vi "Start_Client_Coms.vi"(1 "VI name to run on server":string) -> (2 "LabVIEW application reference":refnum<vi>, 3 "Checked VI name":path, 4 "Local Call":bool)   [LabVIEW 2010]
uses:
  Anemometry/Anemometry Sub Vis/Controls/App_Global.ctl
  Anemometry/Anemometry Sub Vis/Globals/Dynamic_call_global.ph.vi
panel:
  out "Application:Exported VIs In Memory":string[](array[string])
  out "IP & Port No":string
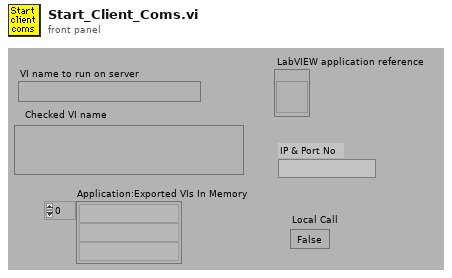
[diagram p1: front panel]
types:
  T1 = typedef "App_Global.ctl" = enum16{"Read Global", "Write to Global", "Initialise Array"}
  T2 = typedef "App_Ref_Cluster.ctl" = cluster{"Server IP & Port No":string, "Application reference":refnum<vi>}
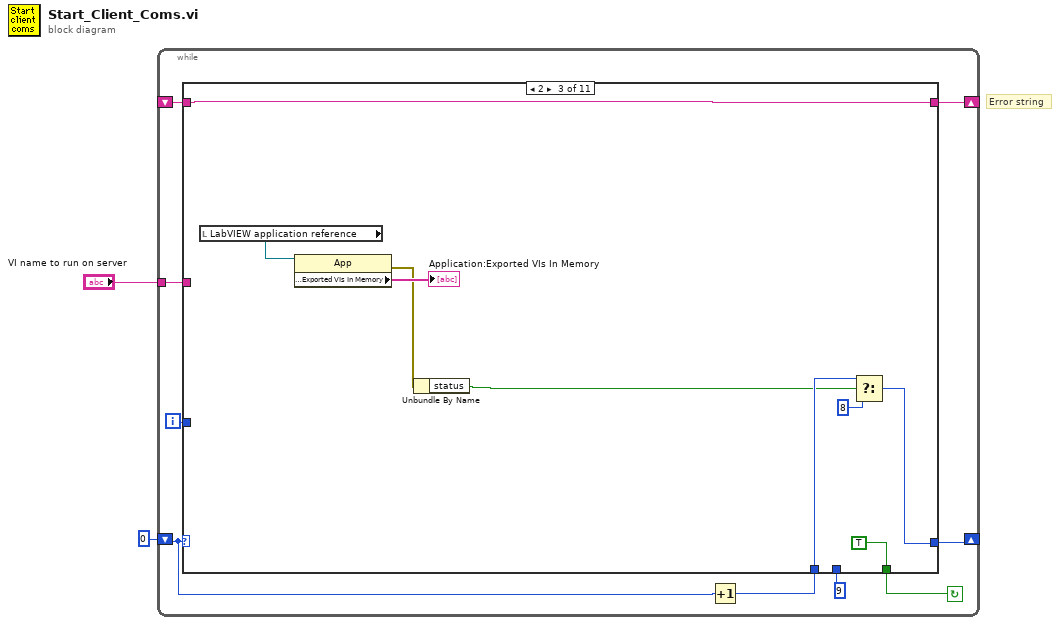
[diagram p0: block diagram]
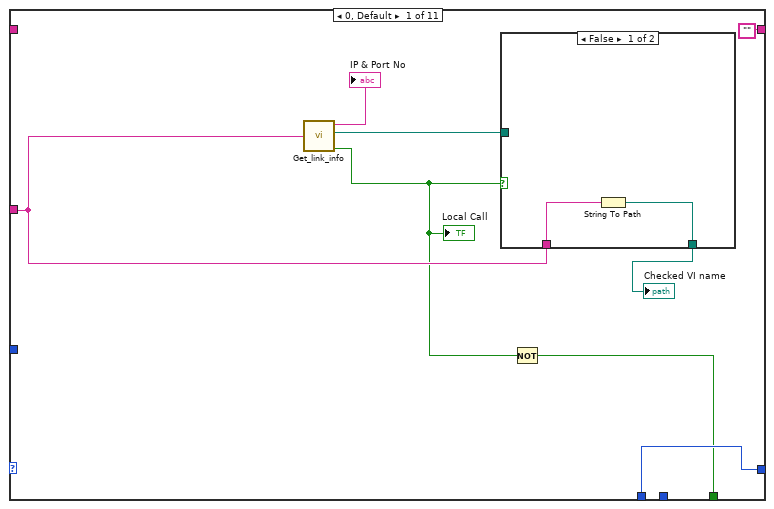
[diagram p2: hidden frame]
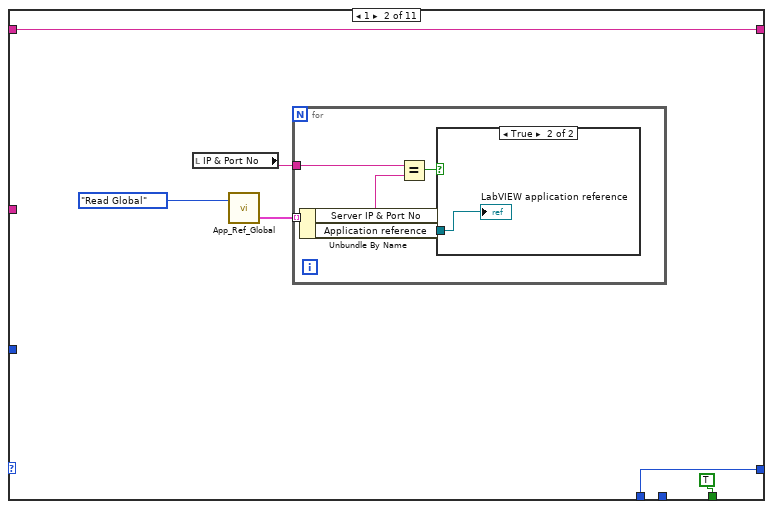
[diagram p4: hidden frame]
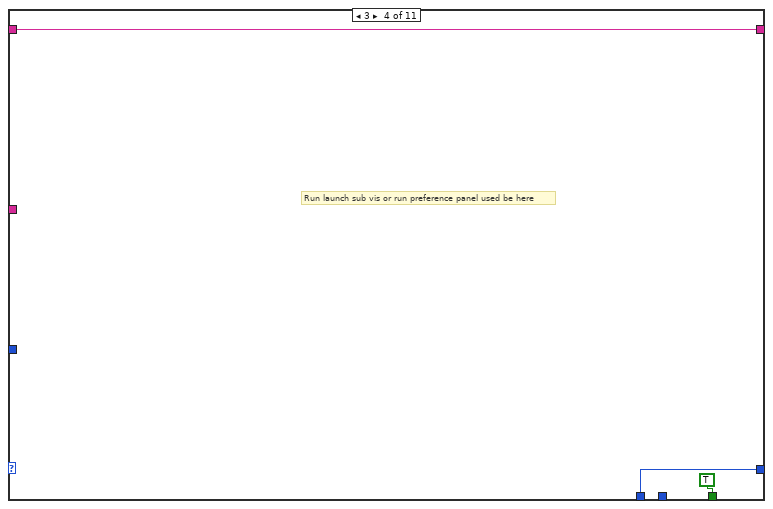
[diagram p6: hidden frame]
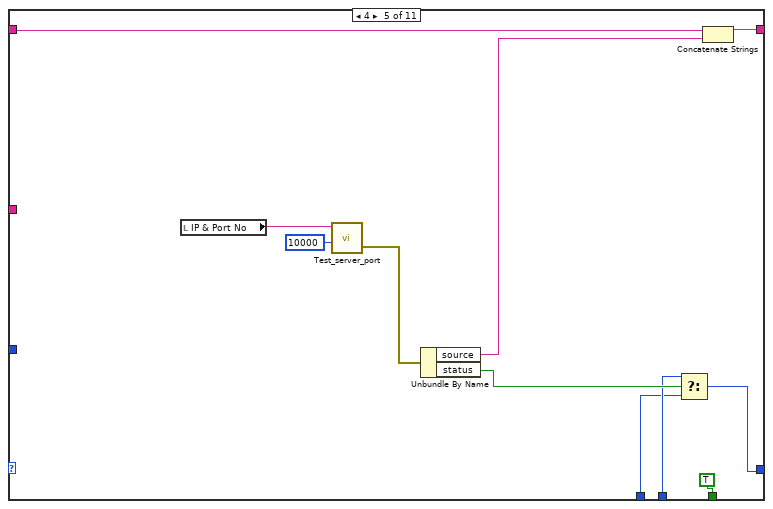
[diagram p7: hidden frame]
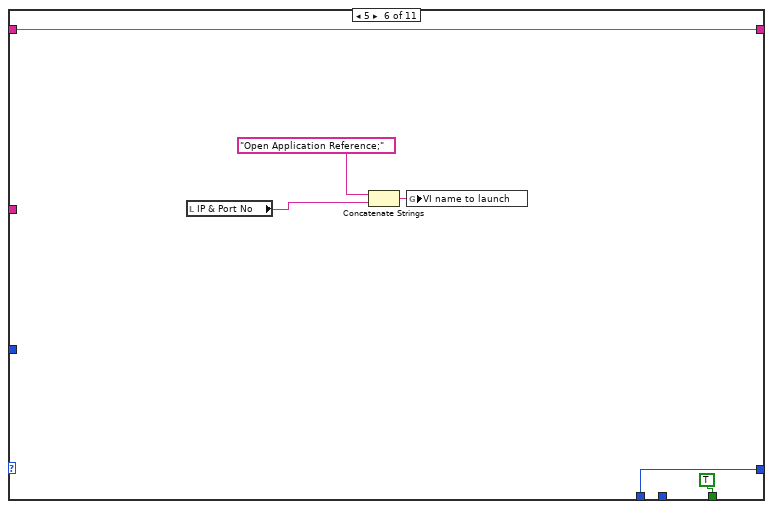
[diagram p8: hidden frame]
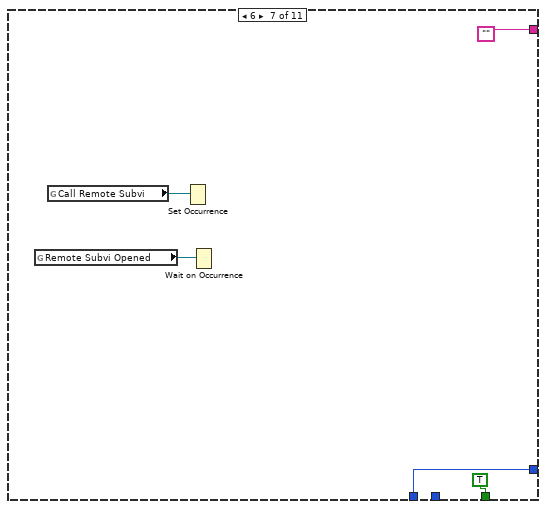
[diagram p9: hidden frame]
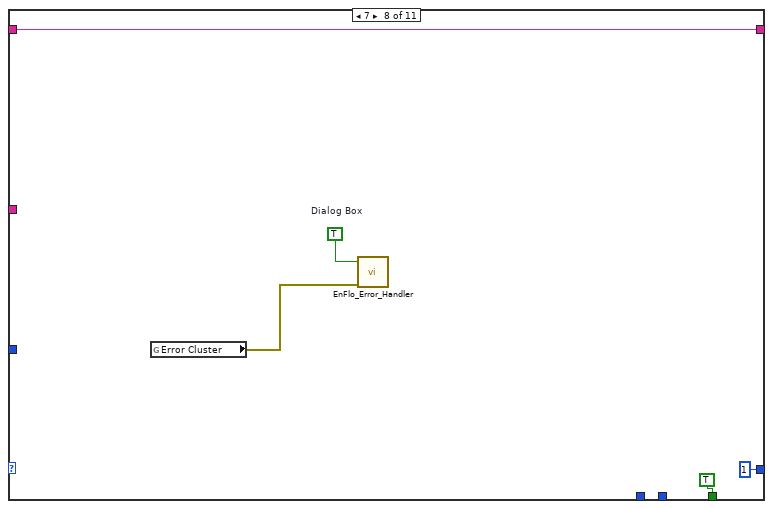
[diagram p10: hidden frame]
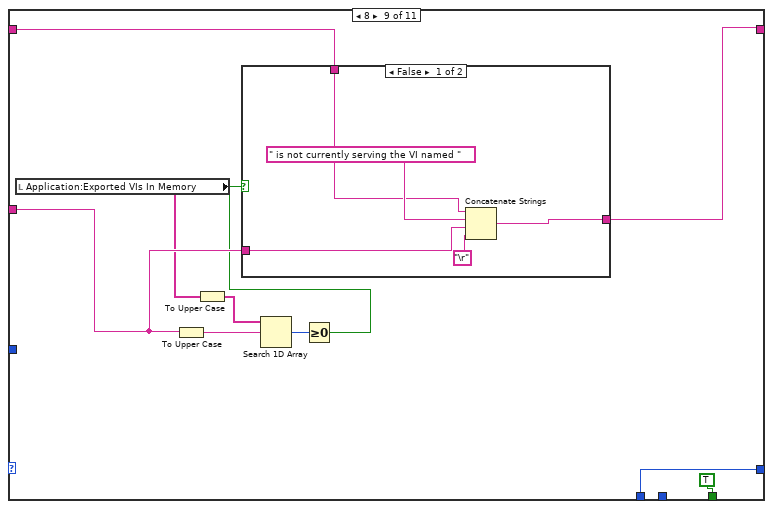
[diagram p11: hidden frame]
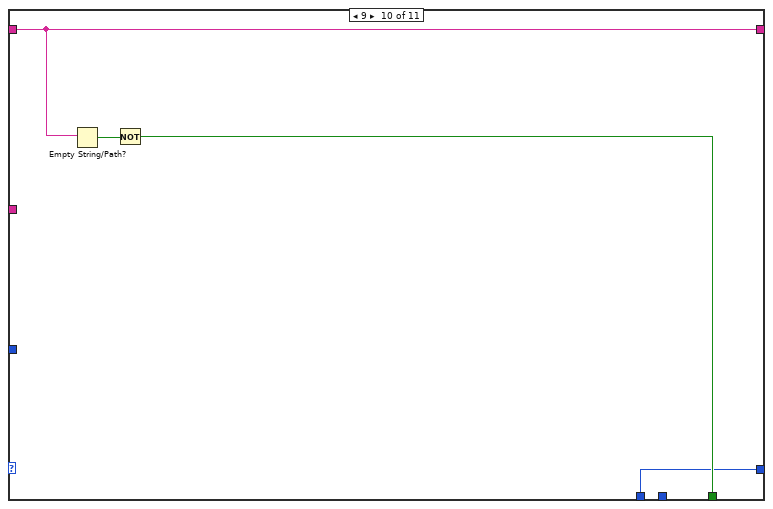
[diagram p13: hidden frame]
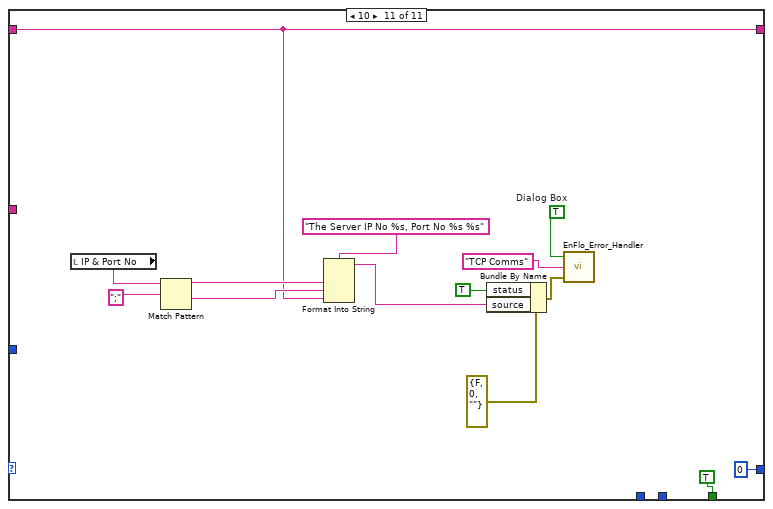
[diagram p14: hidden frame]
diagram:
  # "Error string"
  n1 = while {
    shift-left: _ -> [w4]
    shift-right: [w5] -> _
    shift-left: 0 -> [w9]
    shift-right: [w8] -> _
    tunnel: "VI name to run on server" -> [w10]
    i -> [w6]
    stop <- w11 continue-if-true
    n2 = Increment(x=w9) -> (x+1=w7:i32)
    n3 = case shown="2" w9 {
      tunnel: [w12 TRUE ("status") TRUE ("status") TRUE ("status") TRUE ("status") TRUE ("status") TRUE ("status") TRUE ("status") TRUE ("status") w92 TRUE ("status")] -> w11
      tunnel: w10 -> [w16 _ _ _ _ _ _ _ w83 _ _]
      tunnel: [w18 w26 w40 w46 w47 w62 w64 1 ("f") w76 w91 0 ("f")] -> w8
      tunnel: w7 -> [w18 w26 w41 w46 w48 w62 w64 _ w76 w91 _]
      tunnel: w6 -> [_ _ _ _ _ _ _ _ _ _ _]
      tunnel: ["" w24 w38 w44 w51 w61 "" w70 w74 w90 w98] -> w5
      tunnel: w4 -> [_ w24 w38 w44 w52 w61 _ w70 w75 w90 w98]
      tunnel: 9 ("f") -> [_ _ _ _ w49 _ _ _ _ _ _]
      frame 0, Default {
        n4 = call "Get_link_info.vi"("VI Name"=w16) -> ("Server IP & Port"=→"IP & Port No":string, "Path name"=w14:path, "Local Call?"=w13:bool)  [unwired: 1 out]
        "Local Call" <- w13
        n5 = case shown="False" w13 {
          tunnel: [w20 w22] -> w19
          tunnel: w16 -> [w21 _]
          tunnel: w14 -> [_ w22]
          frame False {
            n6 = String To Path(string=w21) -> (path=w20:path)
          }
          frame True {
          }
        }
        "Checked VI name" <- w19
        n7 = Not(x=w13) -> (.not. x?=w12:bool)
      }
      frame 1 {
        n8 = local read "IP & Port No"() -> (w27:string)
        n9 = call "App_Ref_Global.vi"("Mode"=App_Global."Read Global") -> ("Output Array"=w28:T2[])  [unwired: 1 in, 1 out]
        n10 = for {
          tunnel: w28 -> [w33] mode=indexing
          tunnel: w27 -> [w31]
          n11 = Unbundle By Name(w33) -> ("Server IP & Port No"=w32:string, "Application reference"=w29:refnum<vi>)
          n12 = Equal?(x=w31, y=w32) -> (x = y?=w30:bool)
          n13 = case shown="True" w30 {
            tunnel: w29 -> [_ w34]
            frame False {
            }
            frame True {
              "LabVIEW application reference" <- w34
            }
          }
        }
      }
      frame 2 {
        n14 = local read "LabVIEW application reference"() -> (w43:refnum<vi>)
        n15 = property class="App"(reference=w43) -> (error out=w39:errorcluster, "Application:Exported VIs In Memory"=→"Application:Exported VIs In Memory":string[])  [unwired: 1 in, 1 out]
        n16 = Unbundle By Name(w39) -> ("status"=w36:bool)
        n17 = Select(t=w41, s=w36, f=8) -> (s? t:f=w40:i32)
      }
      frame 3 {
        # "Run launch sub vis or run preference panel used be here"
      }
      frame 4 {
        n18 = local read "IP & Port No"() -> (w56:string)
        n19 = call "Test_server_port.vi"("IP & Port No"=w56, "timeout ms (60000)"=10000) -> ("error out"=w55:errorcluster)  [unwired: 1 in, 3 out]
        n20 = Unbundle By Name(w55) -> ("source"=w53:string, "status"=w50:bool)
        n21 = Select(t=w49, s=w50, f=w48) -> (s? t:f=w47:i32)
        n22 = Concatenate Strings(w52, w53) -> (w51:string)
      }
      frame 5 {
        n23 = local read "IP & Port No"() -> (w59:string)
        n24 = Concatenate Strings("Open Application Reference;", w59) -> (w58:string)
        n25 = global write "Dynamic_call_global.ph.vi" "VI name to launch"(w58) -> ()
      }
      frame 6 {
        n26 = global read "Dynamic_call_global.ph.vi" "Remote Subvi Opened"() -> (w67:refnum<k4>)
        n27 = global read "Dynamic_call_global.ph.vi" "Call Remote Subvi"() -> (w66:refnum<k4>)
        n28 = Set Occurrence(w66) -> ()
        n29 = Wait on Occurrence(2:w67) -> ()  [unwired: 3 out]
      }
      frame 7 {
        w73 = TRUE  # Dialog Box
        n30 = global read "Dynamic_call_global.ph.vi" "Error Cluster"() -> (w72:errorcluster)
        n31 = call "EnFlo_Error_Handler.vi"("error in (no error)"=w72, "Dialog Box (T)"=w73) -> ()  [unwired: 1 in, 3 out]
      }
      frame 8 {
        n32 = local read "Application:Exported VIs In Memory"() -> (w78:string[])
        n33 = To Upper Case(1:w83) -> (0:w82:string)
        n34 = To Upper Case(1:w78) -> (0:w81:string[])
        n35 = Search 1D Array(1D array=w81, element=w82) -> (index of element=w80:i32)  [unwired: 1 out]
        n36 = Greater Or Equal To 0?(x=w80) -> (x >= 0?=w79:bool)
        n37 = case shown="False" w79 {
          tunnel: w83 -> [w87 _]
          tunnel: w75 -> [w86 w89]
          tunnel: [w85 w89] -> w74
          frame False {
            n38 = Concatenate Strings(w86, " is not currently serving the VI named " ("Substring"), w87, "\r") -> (w85:string)
          }
          frame True {
          }
        }
      }
      frame 9 {
        n39 = Empty String/Path?(string/path=w90) -> (empty?=w93:bool)
        n40 = Not(x=w93) -> (.not. x?=w92:bool)
      }
      frame 10 {
        w107 = TRUE  # Dialog Box
        n41 = local read "IP & Port No"() -> (w106:string)
        n42 = Match Pattern(string=w106, regular expression=";") -> (before substring=w103:string, after substring=w102:string)  [unwired: 3 out]
        n43 = Format Into String(format string="The Server IP No %s, Port No %s %s" ("Format String"), w103, w102, w98) -> (resulting string=w97:string)  [unwired: 2 in, 1 out]
        n44 = Bundle By Name(cluster=errorcluster {"status"=FALSE, "code"=0, "source"=""} ("error in (no error)"), "status"=TRUE ("Bundle Element"), "source"=w97) -> (w99:errorcluster)
        n45 = call "EnFlo_Error_Handler.vi"("error in (no error)"=w99, "Error Type"="TCP Comms", "Dialog Box (T)"=w107) -> ()  [unwired: 3 out]
      }
    }
  }
